vi "Go To Starting Command.vi"(8 "error in (no error)":errorcluster, 11 "Command Processor in":refnum<class "Running Command.lvclass">) -> (0 "error out":errorcluster, 3 "State out":refnum<class "State Actor.lvclass">)   [LabVIEW 2014, in "Robot Actor Framework.lvlib" / "Command Processor Actor.lvlib" / "Running Command.lvclass"]
uses:
  Running Command.lvclass
  <vilib>/ni/Actors/State Actor/State Actor/State Actor.lvclass
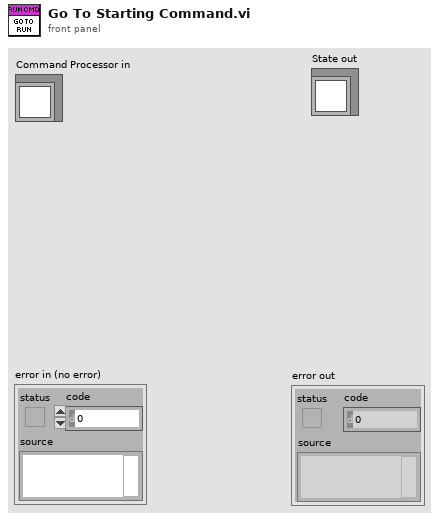
[diagram p1: front panel]
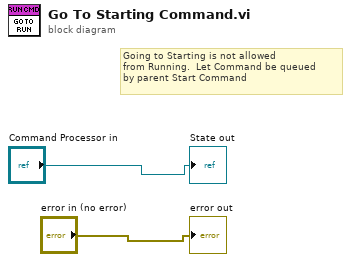
[diagram p0: block diagram]
diagram:
  # "Going to Starting is not allowed \nfrom Running.  Let Command be queued\nby parent Start Command"
  "error out" <- "error in (no error)"
  "State out" <- "Command Processor in"
